vi "New from timestamp.vi"(10 "Type":T1, 11 "Timestamp (now)":timestamp) -> (3 "MsgPackTimestamp out":refnum<class "MsgPackTimestamp.lvclass">)   [LabVIEW 2020, in "MessagePack.lvlib" / "MsgPackTimestamp.lvclass"]
uses:
  MsgPackTimestamp.lvclass
  Type.ctl
  MsgPackTimestamp.lvclass/MsgPackTimestamp.ctl
  <vilib>/LabVIEW Open Source Project/Epoch Date & Time/epoch.UNIX/Epoch.UNIX.lvclass
  C:/Program Files (x86)/National Instruments/LabVIEW 2020/vi.lib/LabVIEW Open Source Project/Epoch Date & Time/epoch/Epoch.lvclass
  <vilib>/LabVIEW Open Source Project/Epoch Date & Time/Get Epoch Time.vi
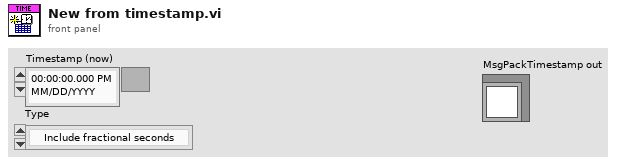
[diagram p1: front panel]
types:
  T1 = typedef "MessagePack.lvlib/MsgPackTimestamp.lvclass/Type.ctl" = enum16{"Include fractional seconds", "Seconds only"}
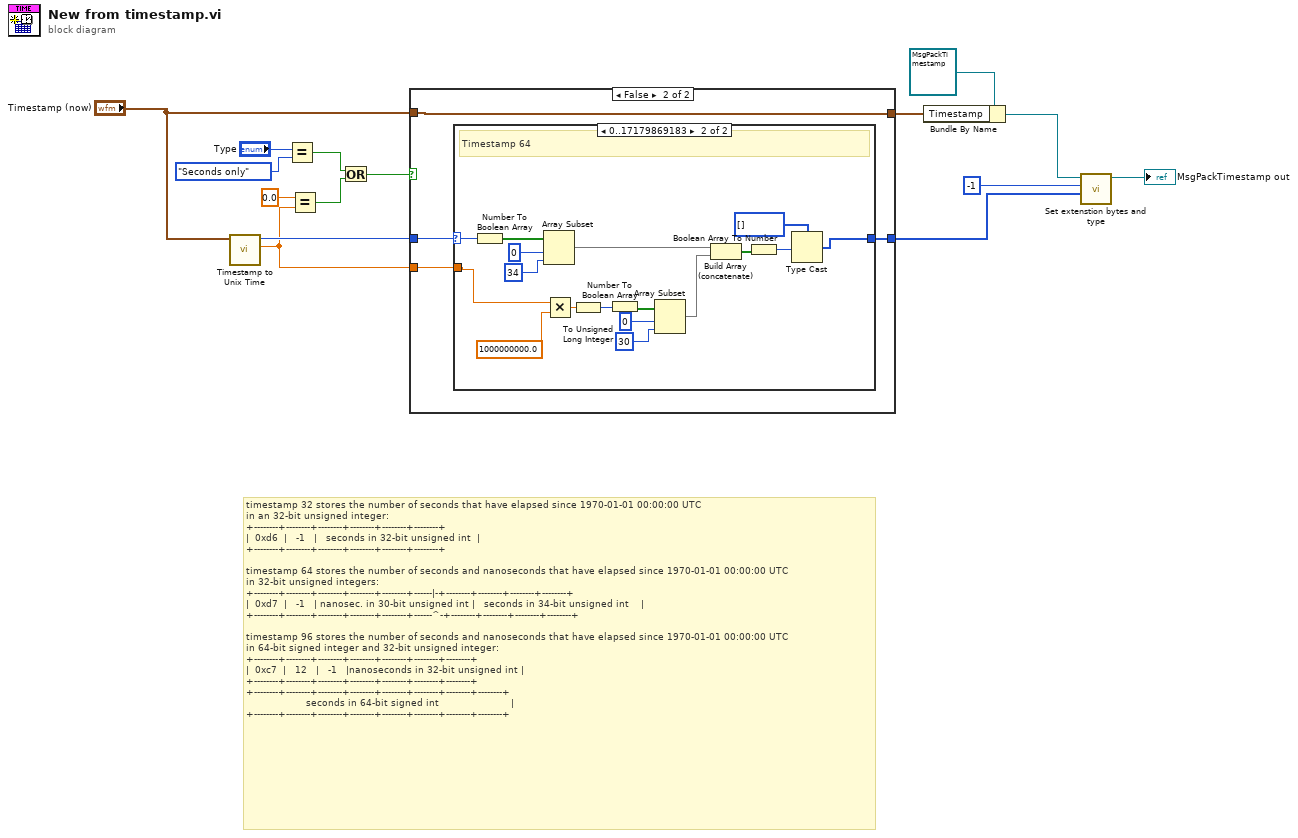
[diagram p0: block diagram]
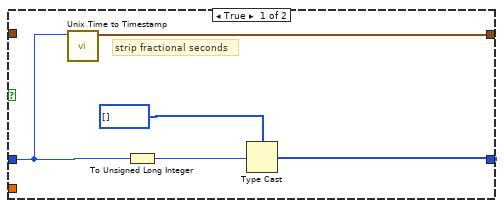
[diagram p2: hidden frame]
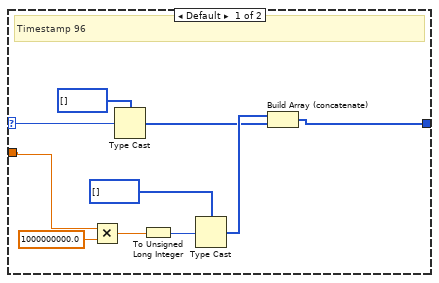
[diagram p3: hidden frame]
diagram:
  # "timestamp 32 stores the number of seconds that have elapsed since 1970-01-01 00:00:00 UTC\nin an 32-bit unsigned integer:\n+--------+--------+--------+--------+--------+--------+\n|  0xd6  |   -1   |   seconds in 32-bit unsigned int  |\n+--------+--------+--------+--------+--------+--------+\n\ntimestamp 64 stores the number of seconds and nanoseconds that have elapsed since 1970-01-01 00:00:00 UTC\nin 32-bit unsigned integers:\n+--------+--------+--------+--------+--------+------|-+--------+--------+--------+--------+\n|  0xd7  |   -1   | nanosec. in 30-bit unsigned int |   seconds in 34-bit unsigned int    |\n+--------+--------+--------+--------+--------+------^-+--------+--------+--------+--------+\n\ntimestamp 96 stores the number of seconds and nanoseconds that have elapsed since 1970-01-01 00:00:00 UTC\nin 64-bit signed integer and 32-bit unsigned integer:\n+--------+--------+--------+--------+--------+--------+--------+\n|  0xc7  |   12   |   -1   |nanoseconds in 32-bit unsigned int |\n+--------+--------+--------+--------+--------+--------+--------+\n+--------+--------+--------+--------+--------+--------+--------+--------+\n                    seconds in 64-bit signed int                        |\n+--------+--------+--------+--------+--------+--------+--------+--------+"
  n1 = call <vilib>:"Timestamp to Unix Time.vi"("Timestamp (now)"="Timestamp (now)") -> ("Fractional Second"=w10:dbl, "Unix Time (s)"=w14:i64)  [unwired: 9 in]
  n2 = Equal?(x="Type", y=Type."Seconds only" ("Type")) -> (x = y?=w11:bool)
  n3 = Equal?(x=0.0, y=w10) -> (x = y?=w8:bool)
  n4 = Or(x=w11, y=w8) -> (x .or. y?=w7:bool)
  n5 = case shown="False" w7 {
    tunnel: w14 -> [w17 w24]
    tunnel: [w18 w22] -> w6
    tunnel: w10 -> [_ w23]
    tunnel: [w16 w21] -> w2
    tunnel: "Timestamp (now)" -> [_ w21]
    frame True {
      # "strip fractional seconds"
      n6 = call <vilib>:"Unix Time to Timestamp.vi"("Unix Time (s)"=w17) -> ("Timestamp"=w16:timestamp)  [unwired: 9 in, 1 out]
      n7 = To Unsigned Long Integer(number=w17) -> (unsigned 32bit integer=w19:u32)
      n8 = Type Cast(type=u8[] [], x=w19) -> (*(type *) &x=w18:u8[])
    }
    frame False {
      n9 = case shown="0..17179869183" w24 {
        selector: w24 -> [w28 w48]
        tunnel: w23 -> [w30 w49]
        tunnel: [w25 w35] -> w22
        frame Default {
          # "Timestamp 96"
          n10 = Multiply(x=w30, y=1000000000.0) -> (x*y=w33:dbl)
          n11 = Type Cast(type=u8[] [], x=w28) -> (*(type *) &x=w26:u8[])
          n12 = To Unsigned Long Integer(number=w33) -> (unsigned 32bit integer=w34:u32)
          n13 = Type Cast(type=u8[] [], x=w34) -> (*(type *) &x=w27:u8[])
          n14 = Build Array (concatenate)(w27, w26) -> (w25:u8[])
        }
        frame 0..17179869183 {
          # "Timestamp 64"
          n15 = Number To Boolean Array(number=w48) -> (Boolean array=w47:bool[])
          n16 = Array Subset(array=w47, index=0, length=34) -> (w40:bool[])
          n17 = Multiply(x=w49, y=1000000000.0) -> (x*y=w51:dbl)
          n18 = To Unsigned Long Integer(number=w51) -> (unsigned 32bit integer=w42:u32)
          n19 = Number To Boolean Array(number=w42) -> (Boolean array=w41:bool[])
          n20 = Array Subset(array=w41, index=0, length=30) -> (w39:bool[])
          n21 = Build Array (concatenate)(w40, w39) -> (w38:bool[])
          n22 = Boolean Array To Number(Boolean array=w38) -> (number=w36:u64)
          n23 = Type Cast(type=u8[] [], x=w36) -> (*(type *) &x=w35:u8[])
        }
      }
    }
  }
  n24 = Bundle By Name(cluster=refnum<class "MsgPackTimestamp.lvclass"> refnum ("MessagePack.lvlib:MsgPackTimestamp.lvclass"), "Timestamp"=w2) -> (w3:refnum<class "MsgPackTimestamp.lvclass">)
  n25 = call-dynamic "Set extenstion bytes and type.vi"("Payload bytes"=w6, "Payload Ext Type"=i8 -1, "MsgPackExt in"=w3) -> ("MsgPackExt out"=→"MsgPackTimestamp out":refnum<class "MsgPackTimestamp.lvclass">)  [unwired: 7 in, 1 out]
